vi "DLPIO20_Digital_IO.vi"(7 "Digital I/O":u8(ring) items=["AN0", "AN1", "AN2", "AN3", "AN4", "AN5", "AN6", "AN7", "AN8", "AN9", "AN10", "AN11", "AN12", "AN13", "RA4", "P5", "P6", "P7", "RB7", "RB6"], 8 "error in (no error)":errorcluster, 9 "Output HI/LOW":bool, 10 "Input/Output":bool, 11 "VISA resource name":refnum<visa-resource-name>) -> (0 "error out":errorcluster, 2 "Input":bool, 3 "VISA resource name out":refnum<visa-resource-name>, 6 "NoError":bool=TRUE)   [LabVIEW 2016, in "DLPIO20_PackedLibrary.lvlib"]
uses:
  DLPIO20_PackedLibrary.lvlib
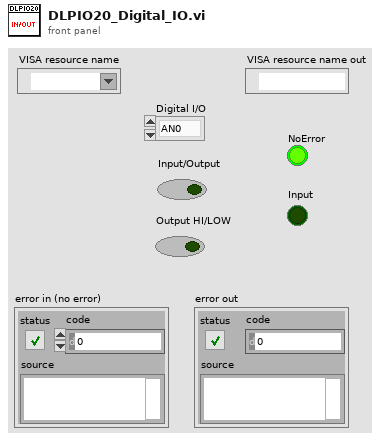
[diagram p1: front panel]
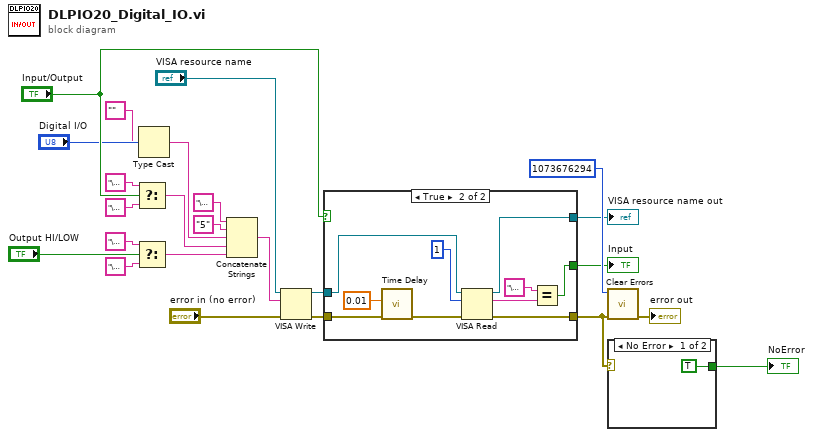
[diagram p0: block diagram]
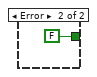
[diagram p2: hidden frame]
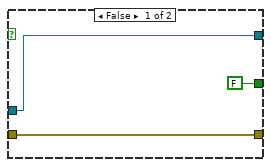
[diagram p3: hidden frame]
diagram:
  n1 = Select(t="\u0001" ("string"), s="Input/Output", f="\u0000" ("string")) -> (s? t:f=w16:string)
  n2 = Select(t="\u0001" ("string"), s="Output HI/LOW", f="\u0000" ("string")) -> (s? t:f=w12:string)
  n3 = Type Cast(type="", x="Digital I/O") -> (*(type *) &x=w5:string)
  n4 = Concatenate Strings("\u0005" ("string"), "5" ("string"), w5, w16, w12) -> (w11:string)
  n5 = VISA Write(VISA resource name="VISA resource name", write buffer=w11, error in (no error)="error in (no error)") -> (VISA resource name out=w9:refnum<visa-resource-name>, error out=w8:errorcluster)  [unwired: 1 out]
  n6 = case shown="True" "Input/Output" {
    tunnel: w9 -> [w26 w34]
    tunnel: w8 -> [w27 w37]
    tunnel: [w27 w35] -> w2
    tunnel: [w26 w32] -> w7
    tunnel: [FALSE w29] -> w6
    frame False {
    }
    frame True {
      n7 = call "Time Delay"("error in (no error)"=w37, "Delay Time (s)"=0.01) -> ("error out"=w36:errorcluster)  [unwired: 9 in]
      n8 = VISA Read(VISA resource name=w34, byte count=u32 1, error in (no error)=w36) -> (VISA resource name out=w32:refnum<visa-resource-name>, read buffer=w31:string, error out=w35:errorcluster)  [unwired: 1 out]
      n9 = Equal?(x="\u0001", y=w31) -> (x = y?=w29:bool)
    }
  }
  "VISA resource name out" <- w7
  "Input" <- w6
  n10 = call <vilib>:"Clear Errors.vi"("error in (no error)"=w2, "specific error code to clear (0: all)"=1073676294) -> ("error out"=→"error out":errorcluster)  [unwired: 4 in, 1 out]
  n11 = case shown="No Error" w2 {
    tunnel: [TRUE FALSE] -> w1
    frame No Error {
    }
    frame Error {
    }
  }
  "NoError" <- w1
